vi "Version String to Cluster.vi"(8 "error in (no error)":errorcluster, 11 "version string":string) -> (0 "error out":errorcluster, 3 "version":T1)   [LabVIEW 2017, in "DSF System Explorer.lvlib"]
uses:
  DSF System Explorer.lvlib
  DSF Core.lvlibp/Typedefs/DSF Version Info.ctl
  <vilib>/Utility/error.llb/whitespace.ctl
  DSF Core.lvlibp
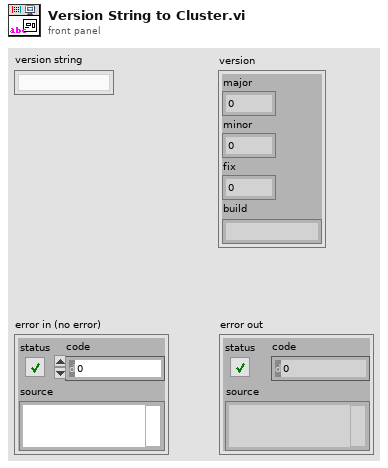
[diagram p1: front panel]
types:
  T1 = typedef "DSF Core.lvlibp/DSF Version Info.ctl" = cluster{"major":u32, "minor":u32, "fix":u32, "build":string}
  T2 = typedef "whitespace.ctl" = u16
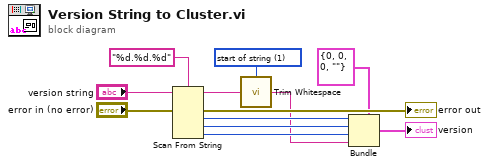
[diagram p0: block diagram]
diagram:
  w6 = T2 1 items=["both", "start of string", "end of string"] ("location (both)")
  n1 = Scan From String(format string="%d.%d.%d", input string="version string", error in="error in (no error)") -> (remaining string=w5:string, error out=→"error out":errorcluster, output 1=w10:i32, output 2=w9:i32, output 3=w8:i32)  [unwired: 4 in, 1 out]
  n2 = call <vilib>:"Trim Whitespace.vi"("string"=w5, "location (both)"=w6) -> ("trimmed string"=w2:string)
  n3 = Bundle(cluster=T1 {"major"=0, "minor"=0, "fix"=0, "build"=""} ("version"), "major"=w10, "minor"=w9, "fix"=w8, "build"=w2) -> (→"version":T1)
